vi "Read Both Fans Fault and State.vi"(8 "error in (no error)":cluster{"状态":bool, "代码":i32, "源":string} caption="错误输入（无错误）", 11 "硬件双风扇输入":refnum<class "HW Dual Fan.lvclass">) -> (0 "error out":cluster{"状态":bool, "代码":i32, "源":string} caption="错误输出", 1 "风扇B故障":bool, 2 "风扇B状态":bool, 3 "风扇A故障":bool, 5 "风扇A状态":bool)   [LabVIEW 2013, in "HW Dual Fan.lvclass"]
uses:
  HW Dual Fan.lvclass
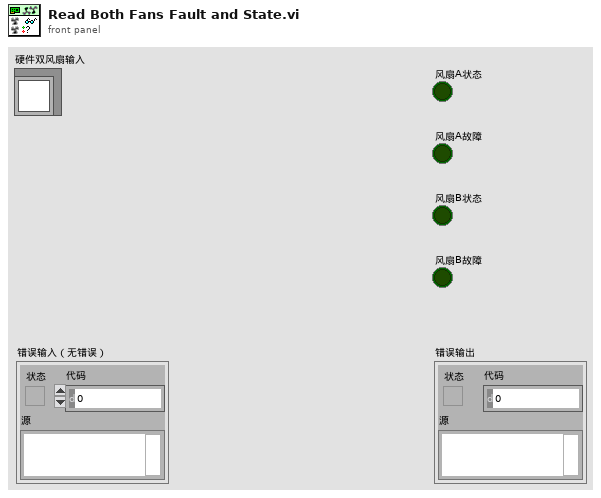
[diagram p1: front panel]
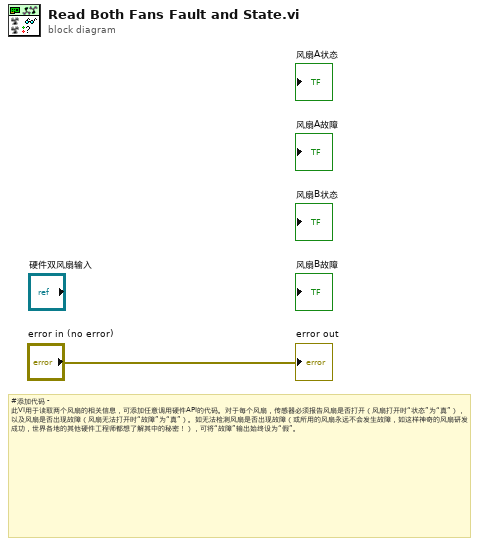
[diagram p0: block diagram]
diagram:
  # "#添加代码 - 此VI用于读取两个风扇的相关信息，可添加任意调用硬件API的代码。对于每个风扇，传感器必须报告风扇是否打开（风扇打开时“状态”为“真”），以及风扇是否出现故障（风扇无法打开时“故障”为“真”）。如无法检测风扇是否出现故障（或所用的风扇永远不会发生故障，如这样神奇的风扇研发成功，世界各地的其他硬件工程师都想了解其中的秘密！），可将“故障”输出始终设为“假”。"
  "error out" <- "error in (no error)"
